vi "RT FIFO.vi"() -> ()   [LabVIEW 2014]
uses:
  <vilib>/Platform/TimedLoop/XDataNode/timing_clust.ctl
  <vilib>/Platform/TimedLoop/XDataNode/nitl_modes.ctl
  <vilib>/Platform/TimedLoop/XDataNode/wakeup.ctl
  <vilib>/Platform/TimedLoop/XDataNode/XDataNode.xnode
  <vilib>/Platform/TimedLoop/XDataNode/XDNodeRunTimeDep.lvlib
panel:
  out "Waveform Chart":dbl(graph)
  in  "Vertical Pointer Slide":dbl(slide) scale=0.0..10.0
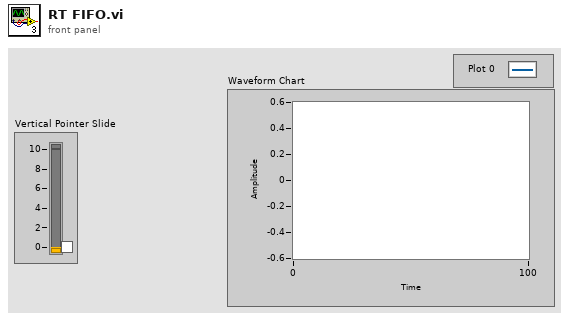
[diagram p1: front panel]
types:
  T1 = typedef "XDNodeRunTimeDep.lvlib/timing_clust.ctl" = cluster{"Expected End [f-1]":u64, "Actual End [f-1]":u64, "Finished Late? [f-1]":bool, "Expected End [i-1]":u64, "Actual End [i-1]":u64, "Finished Late? [i-1]":bool, "Expected Start [i]":u64, "Actual Start [i]":u64, "Expected Start [f]":u64, "Actual Start [f]":u64, "Source Name":string, "Structure Name":string, "Period":i64, "Deadline":i64, "Offset":i64, "Start":i64, "Priority":i32, "Timeout":i32, "Mode":T2, "Wakeup Reason":T3, "Error":errorcluster, "Source Type":string, "Secondary Source Type":string, "Global End Time":u64, "Global Start Time":u64, "Frame Duration":u64, "Iteration Duration":u64, "Assigned CPU":i32, "I/O Scan Engine Mode":u32}
  T2 = typedef "XDNodeRunTimeDep.lvlib/nitl_modes.ctl" = enum32{"No Change", "Process missed periods, maintain original phase", "Discard missed periods, maintain original phase", "Process missed periods, ignore original phase", "Discard missed periods, ignore original phase"}
  T3 = typedef "XDNodeRunTimeDep.lvlib/wakeup.ctl" = enum32{"Normal", "Aborted", "Asynchronous wakeup", "Timing source error", "Timed loop error", "Timeout"}
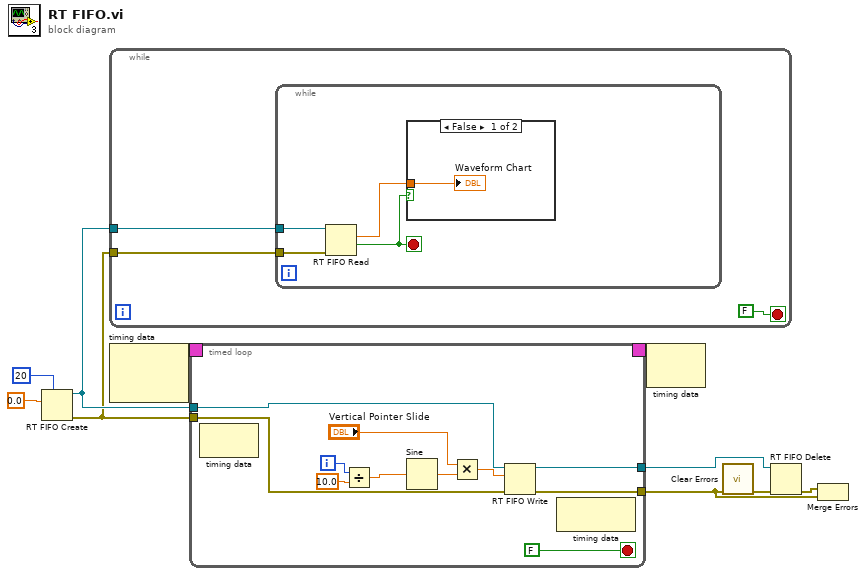
[diagram p0: block diagram]
diagram:
  n1 = RT FIFO Create(1:0.0, 4:u32 20 ("size (10)")) -> (8:w3:refnum<k33>, 11:w2:errorcluster)  [unwired: 6 in, 1 out]
  n2 = while {
    tunnel: w3 -> [w12]
    tunnel: w2 -> [w11]
    stop <- FALSE stop-if-true
    n3 = while {
      tunnel: w12 -> [w16]
      tunnel: w11 -> [w15]
      stop <- w14 stop-if-true
      n4 = RT FIFO Read(0:w16, 3:w15) -> (9:w17:dbl, 10:w14:bool)  [unwired: 2 in, 3 out]
      n5 = case shown="False" w14 {
        tunnel: w17 -> [w18 _]
        frame False {
          "Waveform Chart" <- w18
        }
        frame True {
        }
      }
    }
  }
  n6 = node-c288() -> (w10:T1)  [unwired: 2 in]
  n7 = timed-loop {
    timing: w10 -> [_]
    timing-out: [_] -> w9
    tunnel: w3 -> [w29]
    tunnel: w2 -> [w28]
    tunnel: [w24] -> w5
    tunnel: [w23] -> w4
    i -> [w21]
    stop <- FALSE stop-if-true
    n8 = node-c288() -> ()  [unwired: 1 in, 1 out]
    n9 = Divide(x=w21, y=10.0 ("x")) -> (x/y=w19:dbl)
    n10 = Sine(x=w19) -> (sin(x)=w27:dbl)
    n11 = Multiply(x="Vertical Pointer Slide", y=w27) -> (x*y=w25:dbl)
    n12 = RT FIFO Write(0:w29, 1:w25, 3:w28) -> (8:w23:refnum<k33>, 11:w24:errorcluster)  [unwired: 2 in, 2 out]
    n13 = node-c288() -> ()  [unwired: 1 in, 1 out]
  }
  n14 = node-c288(w9) -> ()  [unwired: 1 out]
  n15 = call <vilib>:"Clear Errors.vi"("error in (no error)"=w5) -> ("error out"=w7:errorcluster)  [unwired: 5 in, 1 out]
  n16 = RT FIFO Delete(0:w4, 3:w7) -> (11:w6:errorcluster)  [unwired: 1 in]
  n17 = Merge Errors(w6, w5) -> ()  [unwired: 1 out]
